vi "Main.vi"(8 "error in (no error)":errorcluster, 11 "ServiceManager in":refnum<class "ServiceManager.lvclass">) -> (0 "error out":errorcluster, 3 "ServiceManager out":refnum<class "ServiceManager.lvclass">)   [LabVIEW 2012, in "ServiceManager.lvclass"]
uses:
  ServiceManager.lvclass
  Murmex/LabVIEW/Murmex/Murmex/status_enum.ctl
  settings_enum.ctl
  ServiceManager.lvclass/ServiceManager.ctl
  Murmex/LabVIEW/Murmex/InitialiseMessage/InitialiseMessage.lvclass
  Murmex/LabVIEW/Murmex/ConfigureMessage/ConfigureMessage.lvclass
  Murmex/LabVIEW/Murmex/InspectMessage/InspectMessage.lvclass
  Murmex/LabVIEW/Murmex/GenericMessage/GenericMessage.lvclass
  Murmex/LabVIEW/Murmex/TerminateMessage/TerminateMessage.lvclass
  Murmex/LabVIEW/Murmex/Murmex/Set configure at initialise.vi
  Murmex/LabVIEW/Murmex/Murmex/Set ID.vi
  Murmex/LabVIEW/Murmex/Murmex/Set VI reference.vi
  Murmex/LabVIEW/Murmex/Murmex/Set log reference.vi
  Murmex/LabVIEW/Murmex/Murmex/Set license required.vi
  Murmex/LabVIEW/Murmex/Murmex/Murmex.lvclass
  Murmex/LabVIEW/Murmex/Message/Message.lvclass
panel:
  in  "button:viewer":bool
  in  "button:licences":bool
  in  "stop":bool
  in  "button:configure":bool
  in  "settings enum":T1 caption="setting"
  in  "Tab Control":enum32{"Components", "Debug", "About"}(tab)
  in  "button:check existence":bool
  in  "components":i32(listbox)
  in  "button:restart_comp":bool
  in  "button:kill_comp":bool
  in  "button:config locally":bool
  out "log":string
  out "status":T2
  out "terminated?":bool
  out "component":refnum<class "ServiceManager.lvclass">
  # "By                        2014"
  # "ServiceManager"
  # "Copyright © 2014 - Distrio\n\nThe ServiceManager allows you to call Murmex executables on your computer. \nWhen another ServiceManager is running on another computer connected to the same RabbitMQ server, you can call a Murmex executable on that computer. Thus setting up a distributed web of Murmex components."
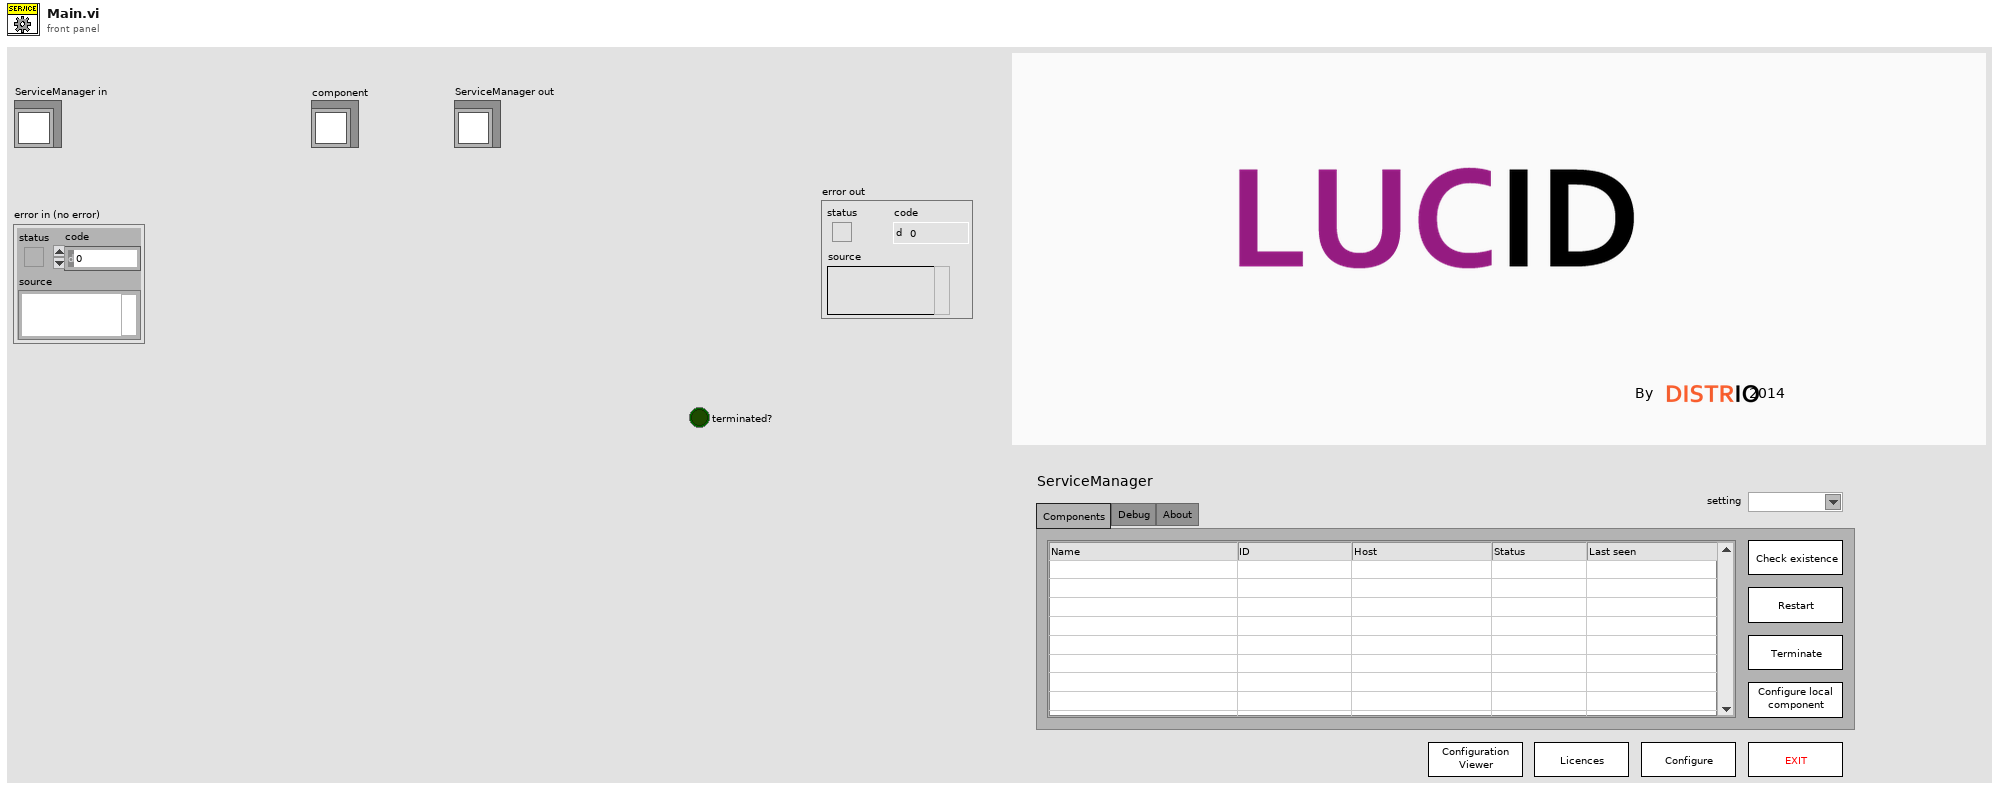
[diagram p1: front panel]
types:
  T1 = typedef "ServiceManager.lvclass/settings_enum.ctl" = string
  T2 = typedef "Murmex.lvlib/Murmex.lvclass/status_enum.ctl" = enum16{"ready", "warning", "error", "shutting down", "initialising"}
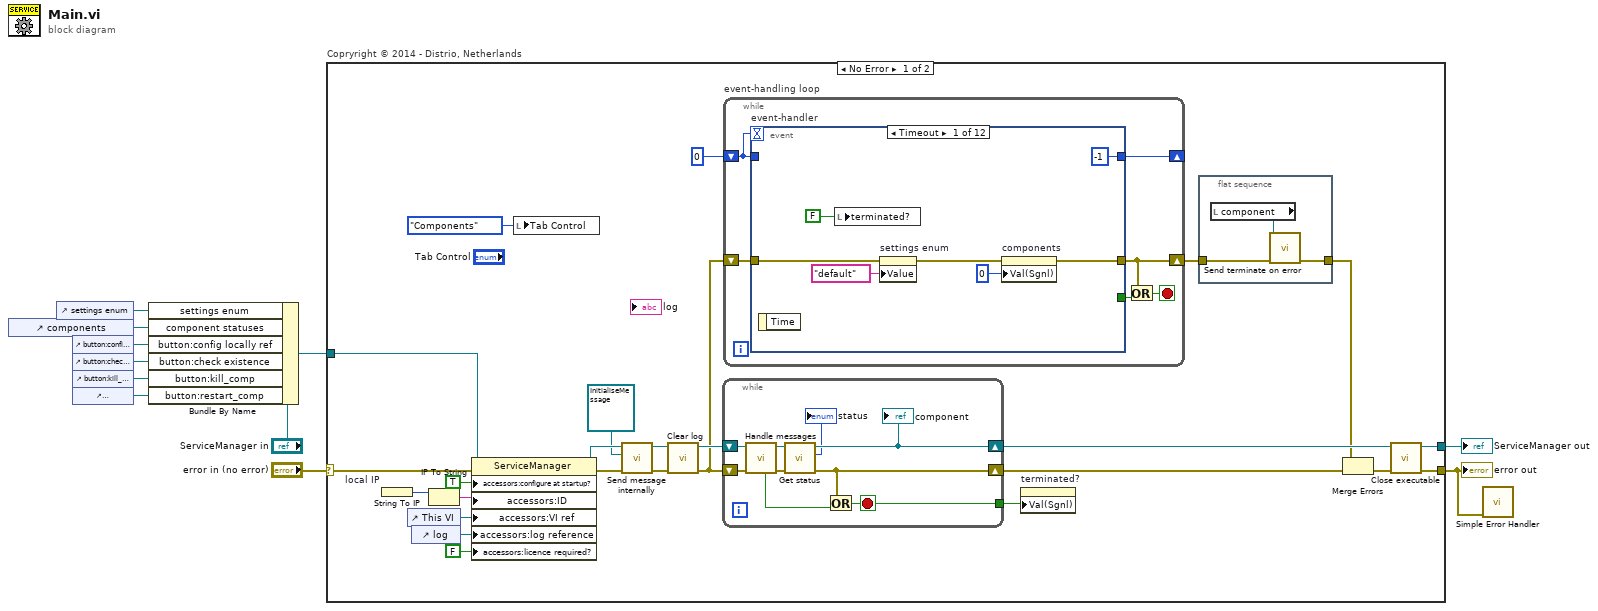
[diagram p0: block diagram]
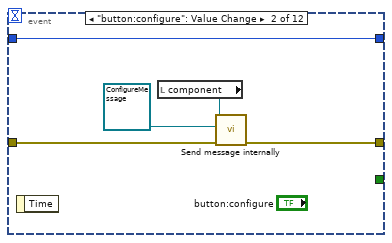
[diagram p2: hidden frame]
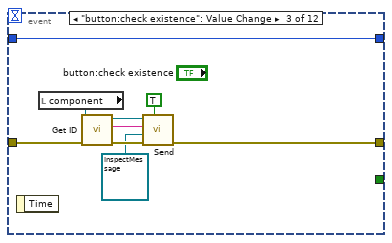
[diagram p3: hidden frame]
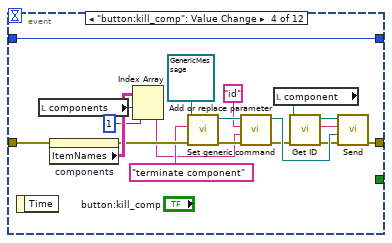
[diagram p4: hidden frame]
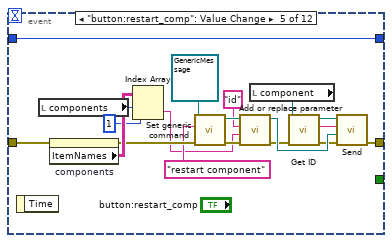
[diagram p5: hidden frame]
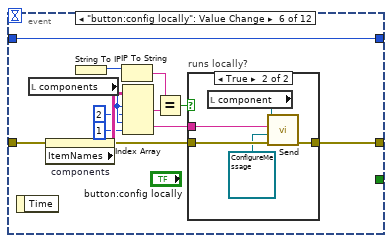
[diagram p6: hidden frame]
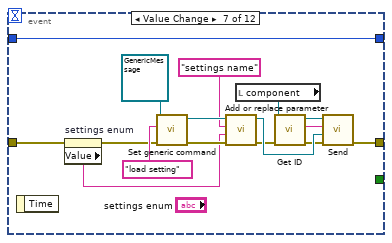
[diagram p8: hidden frame]
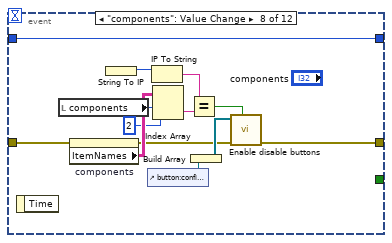
[diagram p9: hidden frame]
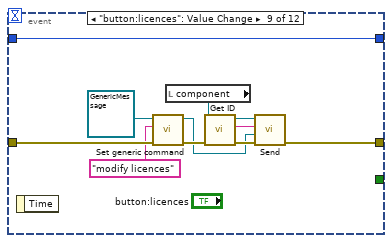
[diagram p10: hidden frame]
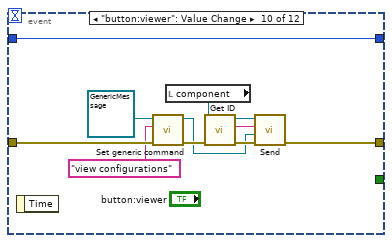
[diagram p11: hidden frame]
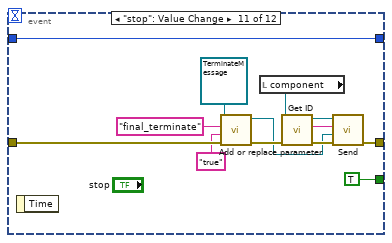
[diagram p12: hidden frame]
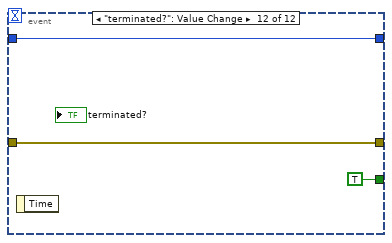
[diagram p13: hidden frame]
diagram:
  n1 = control-ref of="components"() -> (w9:refnum<vi>)
  n2 = control-ref of="settings enum"() -> (w7:refnum<vi>)
  n3 = control-ref of="button:config locally"() -> (w6:refnum<vi>)
  n4 = control-ref of="button:check existence"() -> (w4:refnum<vi>)
  n5 = control-ref of="button:kill_comp"() -> (w3:refnum<vi>)
  n6 = control-ref of="button:restart_comp"() -> (w2:refnum<vi>)
  n7 = Bundle By Name(cluster="ServiceManager in", "settings enum"=w7, "component statuses"=w9, "button:config locally ref"=w6, "button:check existence"=w4, "button:kill_comp"=w3, "button:restart_comp"=w2) -> (w5:refnum<class "ServiceManager.lvclass">)
  n8 = case "Copryright © 2014 - Distrio, Netherlands" shown="No Error" "error in (no error)" {
    selector: "error in (no error)" -> [w12 w201]
    tunnel: [w22 w201] -> w1
    tunnel: [w24 w200] -> w10
    tunnel: w5 -> [w15 w200]
    frame No Error {
      n9 = String To IP "local IP"() -> (0:w36:u32)  [unwired: 1 in]
      n10 = control-ref of="This VI"() -> (w17:refnum<vi>)
      n11 = control-ref of="log"() -> (w28:refnum<vi>)
      n12 = IP To String(2:w36) -> (0:w13:string)  [unwired: 1 in]
      n13 = property class="ServiceManager"(reference=w15, error in=w12, "accessors:configure at startup?"=TRUE ("configure at startup?"), "accessors:ID"=w13, "accessors:VI ref"=w17, "accessors:log reference"=w28, "accessors:licence required?"=FALSE ("licence required?")) -> (reference out=w29:refnum<class "ServiceManager.lvclass">, error out=w16:errorcluster)
      n14 = local write "Tab Control"(enum32{"Components", "Debug", "About"}."Components" ("Tab Control")) -> ()
      n15 = call "Send message internally.vi"("error in (no error)"=w16, "Message"=refnum<class "InitialiseMessage.lvclass"> refnum ("InitialiseMessage.lvclass"), "Murmex in"=w29) -> ("error out"=w27:errorcluster, "Murmex out"=w26:refnum<class "ServiceManager.lvclass">)  [unwired: 7 in]
      n16 = call "Clear log.vi"("error in (no error)"=w27, "MurmexBase in"=w26) -> ("error out"=w31:errorcluster, "MurmexBase out"=w32:refnum<class "ServiceManager.lvclass">)  [unwired: 8 in]
      n17 = while {
        shift-right: [w40] -> w35
        shift-left: w31 -> [w45]
        shift-right: [w47] -> w25
        shift-left: w32 -> [w44]
        tunnel: [w48] -> w34
        stop <- w48 stop-if-true
        n18 = call "Handle messages.vi"("error in (no error)"=w45, "Murmex in"=w44) -> ("error out"=w43:errorcluster, "Murmex out"=w42:refnum<class "ServiceManager.lvclass">, "terminated?"=w41:bool)  [unwired: 7 in]
        n19 = call "Get status.vi"("error in (no error)"=w43, "MurmexBase in"=w42) -> ("error out"=w40:errorcluster, "status"=→"status":T2, "MurmexBase out"=w47:refnum<class "ServiceManager.lvclass">)  [unwired: 6 in, 1 out]
        "component" <- w47
        n20 = Or(x=w40, y=w41) -> (x .or. y?=w48:bool)
      }
      n21 = while "event-handling loop" {
        shift-right: [w53] -> w21
        shift-left: w31 -> [w54]
        shift-right: [w50] -> _
        shift-left: 0 -> [w49]
        stop <- w52 stop-if-true
        n22 = event "event-handler" shown="[0] Timeout" {
          selector: _ -> [_ _ _ _ _ _ _ _ _ _ _ _]
          dyn-events: _ -> [_ _ _ _ _ _ _ _ _ _ _ _]
          timeout: w49 -> [_ _ _ _ _ _ _ _ _ _ _ _]
          tunnel: w54 -> [w56 w62 w73 w93 w112 w124 w147 w151 w165 w176 w188 w199]
          tunnel: [w58 w64 w72 w87 w100 w115 w135 w158 w167 w178 w196 w199] -> w53
          tunnel: [_ _ _ _ _ _ _ _ _ _ TRUE TRUE] -> w51
          tunnel: [-1 w66 w75 w94 w113 w126 w148 w161 w172 w183 w191 w197] -> w50
          tunnel: w49 -> [_ w66 w75 w94 w113 w126 w148 w161 w172 w183 w191 w197]
          event Timeout {
            n23 = event-data() -> ()  [unwired: 1 in, 1 out]
            n24 = local write "terminated?"(FALSE ("terminated?")) -> ()
            n25 = property on="settings enum" class="CmbBox (strict)"(error in=w56, "Value"="default" ("default")) -> (error out=w55:errorcluster)  [unwired: 1 in, 1 out]
            n26 = property on="components" class="MCListbox (strict)"(error in=w55, "Val(Sgnl)"=0 ("statuses")) -> (error out=w58:errorcluster)  [unwired: 1 in, 1 out]
          }
          event "button:configure": Value Change {
            n27 = event-data() -> ()  [unwired: 1 in, 1 out]
            n28 = local read "component"() -> (w65:refnum<class "ServiceManager.lvclass">)
            n29 = call "Send message internally.vi"("error in (no error)"=w62, "Message"=refnum<class "ConfigureMessage.lvclass"> refnum ("ConfigureMessage.lvclass"), "Murmex in"=w65) -> ("error out"=w64:errorcluster)  [unwired: 7 in, 1 out]
          }
          event "button:check existence": Value Change {
            n30 = event-data() -> ()  [unwired: 1 in, 1 out]
            n31 = local read "component"() -> (w74:refnum<class "ServiceManager.lvclass">)
            n32 = call "Get ID.vi"("error in (no error)"=w73, "Murmex in"=w74) -> ("error out"=w68:errorcluster, "component id"=w70:string, "Murmex out"=w71:refnum<class "ServiceManager.lvclass">)  [unwired: 7 in]
            n33 = call "Send.vi"("broadcast? (F)"=TRUE, "error in (no error)"=w68, "Message"=refnum<class "InspectMessage.lvclass"> refnum ("InspectMessage.lvclass"), "recipient"=w70, "Murmex in"=w71) -> ("error out"=w72:errorcluster)  [unwired: 5 in, 1 out]
          }
          event "button:kill_comp": Value Change {
            n34 = event-data() -> ()  [unwired: 1 in, 1 out]
            n35 = local read "components"() -> (w92:i32)
            n36 = property on="components" class="MCListbox (strict)"(error in=w93) -> (error out=w84:errorcluster, "ItemNames"=w91:string[][])  [unwired: 1 in, 1 out]
            n37 = Index Array(array=w91, index (row)=w92, index (col)=1 ("disabled index (col)")) -> (element=w76:string)
            n38 = call "Set generic command.vi"("error in (no error)"=w84, "generic command"="terminate component" ("command string"), "GenericMessage in"=refnum<class "GenericMessage.lvclass"> refnum ("GenericMessage.lvclass")) -> ("error out"=w80:errorcluster, "GenericMessage out"=w82:refnum<class "GenericMessage.lvclass">)  [unwired: 7 in]
            n39 = call "Add or replace parameter.vi"("error in (no error)"=w80, "value"=w76, "name"="id" ("key"), "Message in"=w82) -> ("error out"=w79:errorcluster, "Message out"=w81:refnum<class "GenericMessage.lvclass">)  [unwired: 6 in]
            n40 = local read "component"() -> (w89:refnum<class "ServiceManager.lvclass">)
            n41 = call "Get ID.vi"("error in (no error)"=w79, "Murmex in"=w89) -> ("error out"=w78:errorcluster, "component id"=w86:string, "Murmex out"=w88:refnum<class "ServiceManager.lvclass">)  [unwired: 7 in]
            n42 = call "Send.vi"("error in (no error)"=w78, "Message"=w81, "recipient"=w86, "Murmex in"=w88) -> ("error out"=w87:errorcluster)  [unwired: 6 in, 1 out]
          }
          event "button:restart_comp": Value Change {
            n43 = event-data() -> ()  [unwired: 1 in, 1 out]
            n44 = local read "components"() -> (w111:i32)
            n45 = property on="components" class="MCListbox (strict)"(error in=w112) -> (error out=w99:errorcluster, "ItemNames"=w110:string[][])  [unwired: 1 in, 1 out]
            n46 = Index Array(array=w110, index (row)=w111, index (col)=1 ("disabled index (col)")) -> (element=w95:string)
            n47 = call "Set generic command.vi"("error in (no error)"=w99, "generic command"="restart component" ("command string"), "GenericMessage in"=refnum<class "GenericMessage.lvclass"> refnum ("GenericMessage.lvclass")) -> ("error out"=w102:errorcluster, "GenericMessage out"=w103:refnum<class "GenericMessage.lvclass">)  [unwired: 7 in]
            n48 = call "Add or replace parameter.vi"("error in (no error)"=w102, "value"=w95, "name"="id" ("key"), "Message in"=w103) -> ("error out"=w107:errorcluster, "Message out"=w108:refnum<class "GenericMessage.lvclass">)  [unwired: 6 in]
            n49 = local read "component"() -> (w101:refnum<class "ServiceManager.lvclass">)
            n50 = call "Get ID.vi"("error in (no error)"=w107, "Murmex in"=w101) -> ("error out"=w106:errorcluster, "component id"=w104:string, "Murmex out"=w105:refnum<class "ServiceManager.lvclass">)  [unwired: 7 in]
            n51 = call "Send.vi"("error in (no error)"=w106, "Message"=w108, "recipient"=w104, "Murmex in"=w105) -> ("error out"=w100:errorcluster)  [unwired: 6 in, 1 out]
          }
          event "button:config locally": Value Change {
            n52 = event-data() -> ()  [unwired: 1 in, 1 out]
            n53 = local read "components"() -> (w119:i32)
            n54 = property on="components" class="MCListbox (strict)"(error in=w124) -> (error out=w116:errorcluster, "ItemNames"=w125:string[][])  [unwired: 1 in, 1 out]
            n55 = String To IP ("local IP")() -> (0:w123:u32)  [unwired: 1 in]
            n56 = IP To String(2:w123) -> (0:w122:string)  [unwired: 1 in]
            n57 = Index Array(array=w125, index (row) #1=w119, index (col) #1=2 ("disabled index (col)"), index (row) #2=w119, index (col) #2=1 ("disabled index (col)")) -> (element #1=w121:string, element #2=w114:string)
            n58 = Equal?(x=w122, y=w121) -> (x = y?=w117:bool)
            n59 = case "runs locally?" shown="True" w117 {
              tunnel: w116 -> [w127 w129]
              tunnel: [w127 w132] -> w115
              tunnel: w114 -> [_ w130]
              frame False {
              }
              frame True {
                n60 = local read "component"() -> (w131:refnum<class "ServiceManager.lvclass">)
                n61 = call "Send.vi"("error in (no error)"=w129, "Message"=refnum<class "ConfigureMessage.lvclass"> refnum ("ConfigureMessage.lvclass"), "recipient"=w130, "Murmex in"=w131) -> ("error out"=w132:errorcluster)  [unwired: 6 in, 1 out]
              }
            }
          }
          event Value Change {
            n62 = event-data() -> ()  [unwired: 1 in, 1 out]
            n63 = property on="settings enum" class="CmbBox (strict)"(error in=w147) -> (error out=w134:errorcluster, "Value"=w133:T1)  [unwired: 1 in, 1 out]
            n64 = call "Set generic command.vi"("error in (no error)"=w134, "generic command"="load setting" ("command string"), "GenericMessage in"=refnum<class "GenericMessage.lvclass"> refnum ("GenericMessage.lvclass")) -> ("error out"=w140:errorcluster, "GenericMessage out"=w141:refnum<class "GenericMessage.lvclass">)  [unwired: 7 in]
            n65 = call "Add or replace parameter.vi"("error in (no error)"=w140, "value"=w133, "name"="settings name" ("key"), "Message in"=w141) -> ("error out"=w145:errorcluster, "Message out"=w146:refnum<class "GenericMessage.lvclass">)  [unwired: 6 in]
            n66 = local read "component"() -> (w139:refnum<class "ServiceManager.lvclass">)
            n67 = call "Get ID.vi"("error in (no error)"=w145, "Murmex in"=w139) -> ("error out"=w144:errorcluster, "component id"=w142:string, "Murmex out"=w143:refnum<class "ServiceManager.lvclass">)  [unwired: 7 in]
            n68 = call "Send.vi"("error in (no error)"=w144, "Message"=w146, "recipient"=w142, "Murmex in"=w143) -> ("error out"=w135:errorcluster)  [unwired: 6 in, 1 out]
          }
          event "components": Value Change {
            n69 = event-data() -> ()  [unwired: 1 in, 1 out]
            n70 = local read "components"() -> (w153:i32)
            n71 = property on="components" class="MCListbox (strict)"(error in=w151) -> (error out=w150:errorcluster, "ItemNames"=w157:string[][])  [unwired: 1 in, 1 out]
            n72 = String To IP ("local IP")() -> (0:w156:u32)  [unwired: 1 in]
            n73 = control-ref of="button:config locally"() -> (w160:refnum<vi>)
            n74 = IP To String(2:w156) -> (0:w155:string)  [unwired: 1 in]
            n75 = Index Array(array=w157, index (row)=w153, index (col)=2 ("disabled index (col)")) -> (element=w154:string)
            n76 = Equal?(x=w155, y=w154) -> (x = y?=w149:bool)
            n77 = Build Array(w160) -> (w159:refnum<vi>[])
            n78 = call "Enable disable buttons.vi"("enable?"=w149, "error in (no error)"=w150, "references"=w159) -> ("error out"=w158:errorcluster)  [unwired: 8 in]
          }
          event "button:licences": Value Change {
            n79 = event-data() -> ()  [unwired: 1 in, 1 out]
            n80 = call "Set generic command.vi"("error in (no error)"=w165, "generic command"="modify licences", "GenericMessage in"=refnum<class "GenericMessage.lvclass"> refnum ("GenericMessage.lvclass")) -> ("error out"=w164:errorcluster, "GenericMessage out"=w162:refnum<class "GenericMessage.lvclass">)  [unwired: 7 in]
            n81 = local read "component"() -> (w170:refnum<class "ServiceManager.lvclass">)
            n82 = call "Get ID.vi"("error in (no error)"=w164, "Murmex in"=w170) -> ("error out"=w168:errorcluster, "component id"=w166:string, "Murmex out"=w169:refnum<class "ServiceManager.lvclass">)  [unwired: 7 in]
            n83 = call "Send.vi"("error in (no error)"=w168, "Message"=w162, "recipient"=w166, "Murmex in"=w169) -> ("error out"=w167:errorcluster)  [unwired: 6 in, 1 out]
          }
          event "button:viewer": Value Change {
            n84 = event-data() -> ()  [unwired: 1 in, 1 out]
            n85 = call "Set generic command.vi"("error in (no error)"=w176, "generic command"="view configurations", "GenericMessage in"=refnum<class "GenericMessage.lvclass"> refnum ("GenericMessage.lvclass")) -> ("error out"=w175:errorcluster, "GenericMessage out"=w173:refnum<class "GenericMessage.lvclass">)  [unwired: 7 in]
            n86 = local read "component"() -> (w181:refnum<class "ServiceManager.lvclass">)
            n87 = call "Get ID.vi"("error in (no error)"=w175, "Murmex in"=w181) -> ("error out"=w179:errorcluster, "component id"=w177:string, "Murmex out"=w180:refnum<class "ServiceManager.lvclass">)  [unwired: 7 in]
            n88 = call "Send.vi"("error in (no error)"=w179, "Message"=w173, "recipient"=w177, "Murmex in"=w180) -> ("error out"=w178:errorcluster)  [unwired: 6 in, 1 out]
          }
          event "stop": Value Change {
            n89 = event-data() -> ()  [unwired: 1 in, 1 out]
            n90 = call "Add or replace parameter.vi"("error in (no error)"=w188, "value"="true", "name"="final_terminate", "Message in"=refnum<class "TerminateMessage.lvclass"> refnum ("TerminateMessage.lvclass")) -> ("error out"=w187:errorcluster, "Message out"=w186:refnum<class "TerminateMessage.lvclass">)  [unwired: 6 in]
            n91 = local read "component"() -> (w194:refnum<class "ServiceManager.lvclass">)
            n92 = call "Get ID.vi"("error in (no error)"=w187, "Murmex in"=w194) -> ("error out"=w190:errorcluster, "component id"=w193:string, "Murmex out"=w192:refnum<class "ServiceManager.lvclass">)  [unwired: 7 in]
            n93 = call "Send.vi"("error in (no error)"=w190, "Message"=w186, "recipient"=w193, "Murmex in"=w192) -> ("error out"=w196:errorcluster)  [unwired: 6 in, 1 out]
          }
          event "terminated?": Value Change {
            n94 = event-data() -> ()  [unwired: 1 in, 1 out]
          }
        }
        n95 = Or(x=w53, y=w51) -> (x .or. y?=w52:bool)
      }
      n96 = property on="terminated?" class="Bool (strict)"("Val(Sgnl)"=w34) -> ()  [unwired: 2 in, 2 out]
      n97 = flat-sequence {
        tunnel: w21 -> [w39]
        tunnel: [w38] -> w20
        frame #0 {
          n98 = local read "component"() -> (w37:refnum<class "ServiceManager.lvclass">)
          n99 = call "Send terminate on error.vi"("error in (no error)"=w39, "Murmex in"=w37) -> ("error out"=w38:errorcluster)  [unwired: 8 in, 1 out]
        }
      }
      n100 = Merge Errors(w20, w35) -> (w23:errorcluster)
      n101 = call "Close executable.vi"("error in (no error)"=w23, "MurmexBase in"=w25) -> ("error out"=w22:errorcluster, "MurmexBase out"=w24:refnum<class "ServiceManager.lvclass">)  [unwired: 8 in]
    }
    frame Error {
    }
  }
  "error out" <- w1
  "ServiceManager out" <- w10
  n102 = call <vilib>:"Simple Error Handler.vi"("error in (no error)"=w1) -> ()  [unwired: 4 in, 5 out]
